vi "Process and Filter.vi"(8 "error in (no error)":errorcluster, 11 "SSID Values":T1[](array[typedef])=[{"SSID"="Network", "Pswd?"=FALSE, "Hide?"=FALSE}, {"SSID"="MONU_SIGN_HUB", "Pswd?"=FALSE, "Hide?"=FALSE}, {"SSID"="UHS-GUEST", "Pswd?"=FALSE, "Hide?"=FALSE}, {"SSID"="UHS", "Pswd?"=FALSE, "Hide?"=FALSE}, {"SSID"="MB", "Pswd?"=FALSE, "Hide?"=FALSE}, {"SSID"="MYCAR6741", "Pswd?"=FALSE, "Hide?"=FALSE}, {"SSID"="Justinƒ?Ts", "Pswd?"=FALSE, "Hide?"=FALSE}, {"SSID"="InDemand", "Pswd?"=TRUE, "Hide?"=FALSE}, {"SSID"="RTC-Transit-VLAN", "Pswd?"=FALSE, "Hide?"=FALSE}]) -> (0 "error out":errorcluster, 3 "Results":string[](array[string]))   [LabVIEW 2024]
uses:
  Controls/Network.ctl
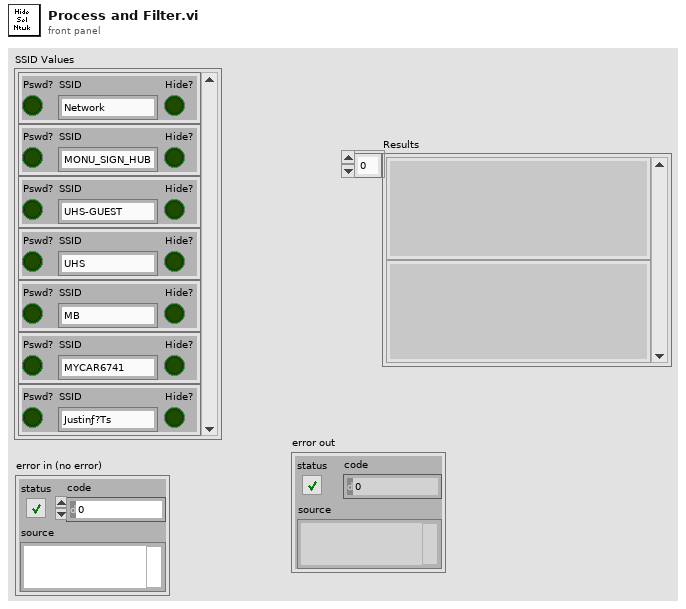
[diagram p1: front panel]
types:
  T1 = typedef "Network.ctl" = cluster{"SSID":string, "Pswd?":bool, "Hide?":bool}
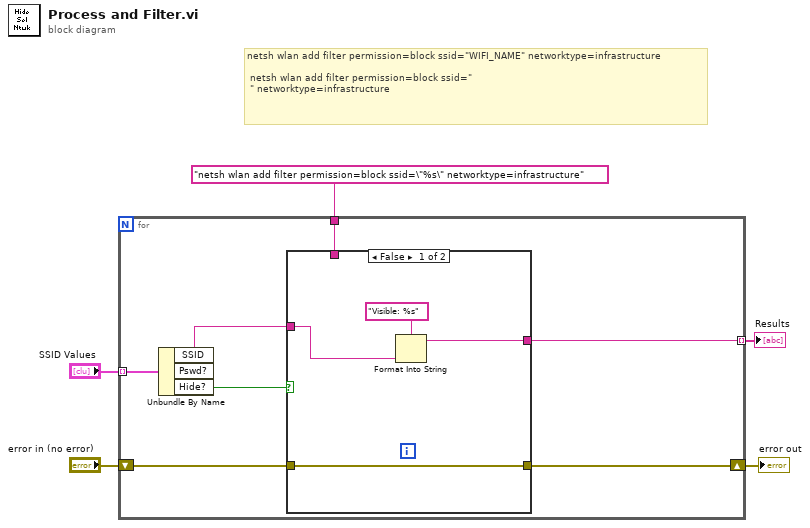
[diagram p0: block diagram]
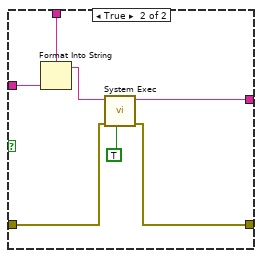
[diagram p2: hidden frame]
diagram:
  # "netsh wlan add filter permission=block ssid=\"WIFI_NAME\" networktype=infrastructure\n\n\tnetsh wlan add filter permission=block ssid=\"\n\t\" networktype=infrastructure"
  n1 = for {
    tunnel: "SSID Values" -> [w12] mode=indexing
    shift-right: [w9] -> w3
    shift-left: "error in (no error)" -> [w10]
    tunnel: "netsh wlan add filter permission=block ssid=\"%s\" networktype=infrastructure" -> [w8]
    tunnel: [w6] -> w1 mode=indexing
    n2 = Unbundle By Name(w12) -> ("SSID"=w7:string, "Hide?"=w11:bool)  [unwired: 1 out]
    n3 = case shown="False" w11 {
      tunnel: w10 -> [w16 w23]
      tunnel: [w16 w22] -> w9
      tunnel: w8 -> [_ w21]
      tunnel: w7 -> [w14 w20]
      tunnel: [w13 w18] -> w6
      frame False {
        n4 = Format Into String(format string="Visible: %s", w14) -> (resulting string=w13:string)  [unwired: 2 in, 1 out]
      }
      frame True {
        n5 = Format Into String(format string=w21, w20) -> (resulting string=w19:string)  [unwired: 2 in, 1 out]
        n6 = call <vilib>:"System Exec.vi"("run minimized? (F)"=TRUE, "error in (no error)"=w23, "command line"=w19) -> ("error out"=w22:errorcluster, "standard output"=w18:string)  [unwired: 5 in, 2 out]
      }
    }
  }
  "error out" <- w3
  "Results" <- w1
